vi "GetInt32Be.vi"(4 "error in (no error)":errorcluster caption="错误输入（无错误）", 7 "refnum in":refnum<file>) -> (0 "error out":errorcluster caption="错误输出", 2 "int32":i32, 3 "refnum out":refnum<file>)   [LabVIEW 2016]
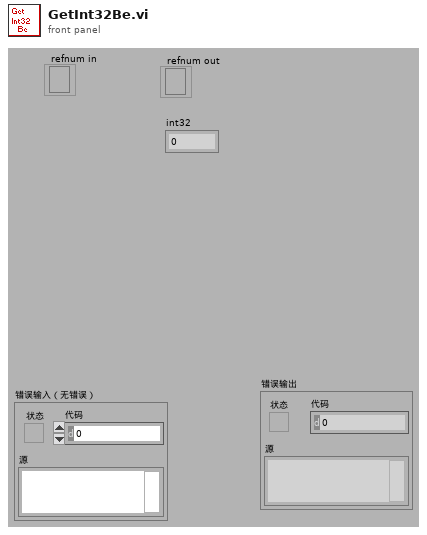
[diagram p1: front panel]
types:
  T1 = enum16{"big-endian, network order", "native, host order", "little-endian"}
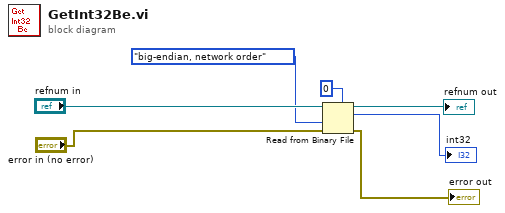
[diagram p0: block diagram]
diagram:
  n1 = Read from Binary File(5:0, 8:"error in (no error)", 9:T1."big-endian, network order" ("字节顺序(0:big-endian, network order)"), 11:"refnum in") -> (0:→"error out":errorcluster, 2:→"int32":i32, 3:→"refnum out":refnum<file>)  [unwired: 3 out]
